vi "vector.vi"(5 "thiccness":sgl=1.0, 6 "style":enum16{"Round", "Square"}(ring), 7 "Color":u32(colorbox)=16711680, 9 "Length X":sgl=10.0, 11 "Name":string) -> (0 "error out":errorcluster, 3 "SceneObject out":refnum<vi>)   [LabVIEW 2022 SP3]
uses:
  <vilib>/picture/3D Picture Control/Object/Create Object (name).vi
  <vilib>/picture/3D Picture Control/Object/Create Object (drawable).vi
  <vilib>/picture/3D Picture Control/Object/Add Object (no reference).vi
  <vilib>/picture/3D Picture Control/NI_3D Picture Control.lvlib
panel:
  out "3D Picture":refnum<vi>(3d-picture)
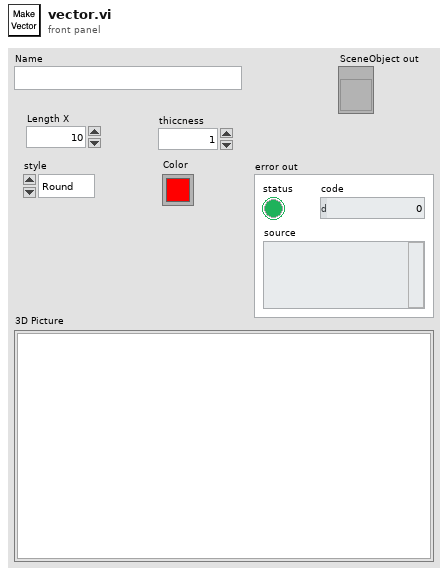
[diagram p1: front panel]
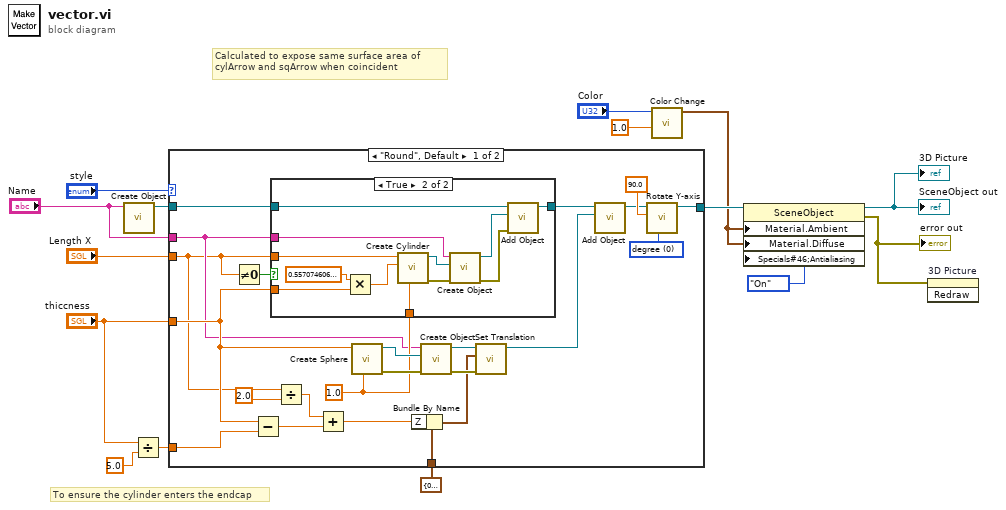
[diagram p0: block diagram]
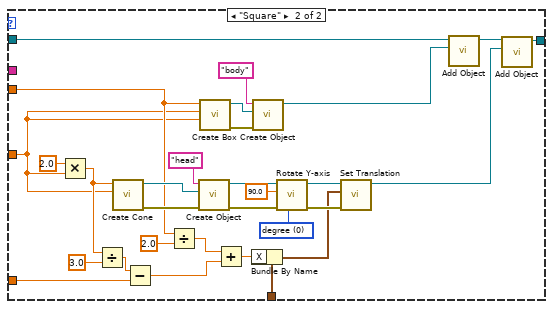
[diagram p3: hidden frame]
diagram:
  # "Calculated to expose same surface area of cylArrow and sqArrow when coincident"
  # "To ensure the cylinder enters the endcap"
  n1 = call-poly <vilib>:"Create Object.vi"("Name"="Name") -> ("Scene:New Object"=w8:refnum<vi>)  [unwired: 9 in, 1 out]
  n2 = Divide(x="thiccness", y=sgl 5.0) -> (x/y=w4:sgl)
  n3 = case shown="\"Round\", Default" "style" {
    tunnel: "thiccness" -> [w20 w55]
    tunnel: "Length X" -> [w16 w61]
    tunnel: cluster{"X":sgl, "Y":sgl, "Z":sgl} {"X"=0.0, "Y"=0.0, "Z"=0.0} ("Translation") -> [w29 w71]
    tunnel: w8 -> [w27 w67]
    tunnel: [w25 w65] -> w7
    tunnel: w4 -> [w19 w54]
    tunnel: "Name" -> [w18 _]
    frame "Round", Default {
      w38 = u16 0 items=["degree", "radians"] ("angle unit")
      w34 = sgl 1.0 ("Detail")
      n4 = Not Equal To 0?(x=w16) -> (x != 0?=w17:bool)
      n5 = Subtract(x=w20, y=w19) -> (x-y=w21:sgl)
      n6 = case shown="True" w17 {
        tunnel: w34 -> [_ w47]
        tunnel: w27 -> [w39 w45]
        tunnel: [w39 w44] -> w26
        tunnel: w16 -> [_ w42]
        tunnel: w20 -> [_ w41]
        tunnel: w18 -> [_ w40]
        frame False {
        }
        frame True {
          n7 = Multiply(x=sgl 0.5570746 ("Radius"), y=w41) -> (x*y=w48:sgl)
          n8 = call <vilib>:"Create Cylinder.vi"("Detail"=w47, "Radius"=w48, "Height"=w42) -> ("error out"=w50:errorcluster, "New Cylinder Refnum"=w51:refnum<vi>)  [unwired: 7 in]
          n9 = call-poly <vilib>:"Create Object.vi"("error in (no error)"=w50, "Geometry"=w51, "Name"=w40) -> ("error out"=w43:errorcluster, "Scene:New Object"=w46:refnum<vi>)  [unwired: 7 in]
          n10 = call-poly <vilib>:"Add Object.vi"("error in (no error)"=w43, "New Object In"=w46, "Scene Object In"=w45) -> ("Scene Object Out"=w44:refnum<vi>)  [unwired: 7 in, 1 out]
        }
      }
      n11 = Divide(x=w16, y=sgl 2.0) -> (x/y=w24:sgl)
      n12 = Add(x=w24, y=w21) -> (x+y=w23:sgl)
      n13 = call <vilib>:"Create Sphere.vi"("Detail"=w34, "Radius"=w20) -> ("error out"=w35:errorcluster, "New Sphere Refnum"=w36:refnum<vi>)  [unwired: 8 in]
      n14 = Bundle By Name(cluster=w29, "Z"=w23) -> (w28:cluster{"X":sgl, "Y":sgl, "Z":sgl})
      n15 = call-poly <vilib>:"Create Object.vi"("error in (no error)"=w35, "Geometry"=w36, "Name"=w18) -> ("error out"=w33:errorcluster, "Scene:New Object"=w32:refnum<vi>)  [unwired: 7 in]
      n16 = call <vilib>:"Set Translation.vi"("error in (no error)"=w33, "Translation"=w28, "Scene Object"=w32) -> ("Translated Object"=w31:refnum<vi>)  [unwired: 7 in, 1 out]
      n17 = call-poly <vilib>:"Add Object.vi"("New Object In"=w31, "Scene Object In"=w26) -> ("Scene Object Out"=w30:refnum<vi>)  [unwired: 8 in, 1 out]
      n18 = call <vilib>:"Rotate Y-axis.vi"("angle unit"=w38, "angle"=90.0, "Scene Object In"=w30) -> ("Scene Object Out"=w25:refnum<vi>)  [unwired: 7 in, 1 out]
    }
    frame "Square" {
      w80 = u16 0 items=["degree", "radians"] ("angle unit")
      n19 = Multiply(x=sgl 2.0 ("y"), y=w55) -> (x*y=w57:sgl)
      n20 = Divide(x=w57, y=sgl 3.0 ("y 2")) -> (x/y=w60:sgl)
      n21 = call <vilib>:"Create Cone.vi"("Radius"=w55, "Height"=w57) -> ("error out"=w76:errorcluster, "New Cone Refnum"=w77:refnum<vi>)  [unwired: 8 in]
      n22 = Subtract(x=w60, y=w54) -> (x-y=w56:sgl)
      n23 = Divide(x=w61, y=sgl 2.0) -> (x/y=w63:sgl)
      n24 = call-poly <vilib>:"Create Object.vi"("error in (no error)"=w76, "Geometry"=w77, "Name"="head") -> ("error out"=w81:errorcluster, "Scene:New Object"=w79:refnum<vi>)  [unwired: 7 in]
      n25 = call <vilib>:"Create Box.vi"("Length Z"=w55, "Length Y"=w55, "Length X"=w61) -> ("error out"=w75:errorcluster, "New Box Refnum"=w69:refnum<vi>)  [unwired: 7 in]
      n26 = Add(x=w63, y=w56) -> (x+y=w58:sgl)
      n27 = Bundle By Name(cluster=w71, "X"=w58) -> (w70:cluster{"X":sgl, "Y":sgl, "Z":sgl})
      n28 = call-poly <vilib>:"Create Object.vi"("error in (no error)"=w75, "Geometry"=w69, "Name"="body") -> ("Scene:New Object"=w68:refnum<vi>)  [unwired: 7 in, 1 out]
      n29 = call <vilib>:"Rotate Y-axis.vi"("angle unit"=w80, "error in (no error)"=w81, "angle"=90.0, "Scene Object In"=w79) -> ("error out"=w73:errorcluster, "Scene Object Out"=w72:refnum<vi>)  [unwired: 6 in]
      n30 = call <vilib>:"Set Translation.vi"("error in (no error)"=w73, "Translation"=w70, "Scene Object"=w72) -> ("Translated Object"=w74:refnum<vi>)  [unwired: 7 in, 1 out]
      n31 = call-poly <vilib>:"Add Object.vi"("New Object In"=w68, "Scene Object In"=w67) -> ("Scene Object Out"=w66:refnum<vi>)  [unwired: 8 in, 1 out]
      n32 = call-poly <vilib>:"Add Object.vi"("New Object In"=w74, "Scene Object In"=w66) -> ("Scene Object Out"=w65:refnum<vi>)  [unwired: 8 in, 1 out]
    }
  }
  n33 = call <vilib>:"Color Change.vi"("Alpha"=1.0, "Color"="Color") -> ("RGBA"=w3:cluster{"R":sgl, "G":sgl, "B":sgl, "A":sgl})  [unwired: 9 in]
  n34 = property class="SceneObject"(reference=w7, "Material.Ambient"=w3, "Material.Diffuse"=w3, "Specials#46;Antialiasing"=enum16{"Inherit Value", "Off", "On"}."On" ("Specials:Anti-aliasing")) -> (reference out=→"SceneObject out" →"3D Picture":refnum<vi>, error out=w10:errorcluster)  [unwired: 1 in]
  "error out" <- w10
  n35 = invoke on="3D Picture" class="SceneGraphDisp (strict)" method="Redraw"(error in=w10) -> ()  [unwired: 2 in, 3 out]
